vi "window_graph get_calc_region.vi"(9 "mouse up pos":cluster{"X":dbl, "Y":dbl}, 10 "mouse down pos":cluster{"X":dbl, "Y":dbl}, 11 "element":cluster{dbl[], sgl[]}) -> (1 "valid":bool, 2 "region data":cluster{"X":dbl, "Y":dbl}[](array[cluster]), 3 "limit data":cluster{"X":dbl, "Y":dbl}[](array[cluster]))   [LabVIEW 2018]
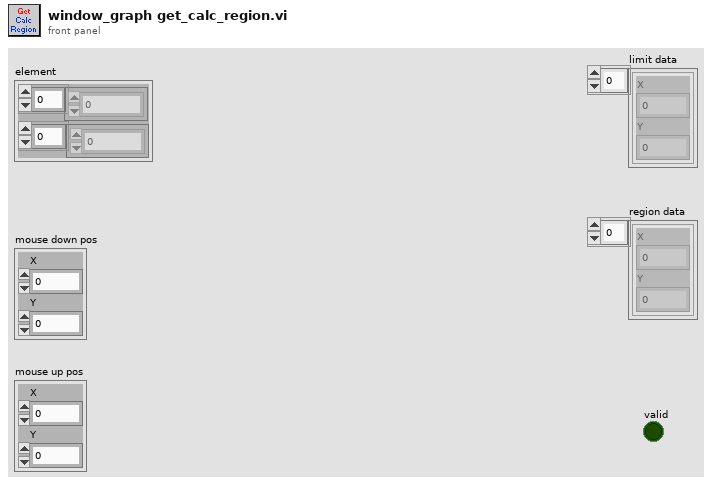
[diagram p1: front panel]
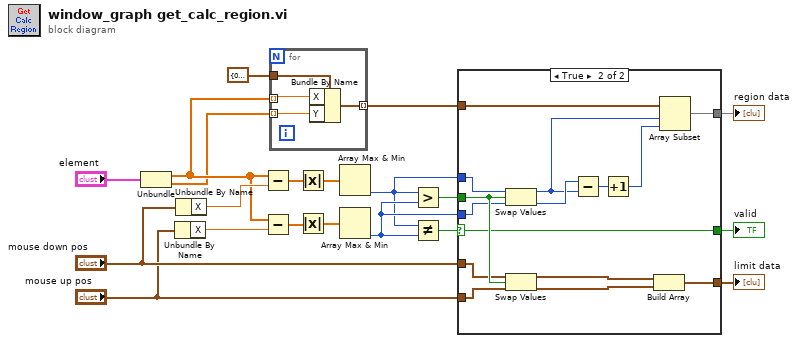
[diagram p0: block diagram]
diagram:
  n1 = Unbundle("element") -> (w13:dbl[], w12:sgl[])
  n2 = Unbundle By Name("mouse up pos") -> ("X"=w19:dbl)
  n3 = Unbundle By Name("mouse down pos") -> ("X"=w20:dbl)
  n4 = Subtract(x=w13, y=w20) -> (x-y=w18:dbl[])
  n5 = Subtract(x=w13, y=w19) -> (x-y=w17:dbl[])
  n6 = for {
    tunnel: cluster{"X":dbl, "Y":dbl} {"X"=0.0, "Y"=0.0} ("mouse down pos") -> [w24]
    tunnel: w13 -> [w23] mode=indexing
    tunnel: w12 -> [w22] mode=indexing
    tunnel: [w21] -> w4 mode=indexing
    n7 = Bundle By Name(cluster=w24, "X"=w23, "Y"=w22) -> (w21:cluster{"X":dbl, "Y":dbl})
  }
  n8 = Absolute Value(x=w18) -> (abs(x)=w16:dbl[])
  n9 = Absolute Value(x=w17) -> (abs(x)=w15:dbl[])
  n10 = Array Max & Min(array=w16) -> (min index (indices)=w5:i32)  [unwired: 3 out]
  n11 = Array Max & Min(array=w15) -> (min index (indices)=w6:i32)  [unwired: 3 out]
  n12 = Greater?(x=w5, y=w6) -> (0:w9:bool)
  n13 = Not Equal?(x=w5, y=w6) -> (x != y?=w10:bool)
  n14 = case shown="True" w10 {
    selector: w10 -> [w25 w30]
    tunnel: w9 -> [_ w40]
    tunnel: "mouse down pos" -> [_ w39]
    tunnel: "mouse up pos" -> [_ w38]
    tunnel: w6 -> [_ w36]
    tunnel: w5 -> [_ w37]
    tunnel: w4 -> [_ w29]
    tunnel: [_ w32] -> w1
    tunnel: [_ w31] -> w2
    tunnel: [w25 w30] -> w3
    frame False {
    }
    frame True {
      n15 = Swap Values(12:w37, 13:w40, 14:w36) -> (1:w28:i32, 3:w35:i32)
      n16 = Swap Values(12:w39, 13:w40, 14:w38) -> (1:w34:cluster{"X":dbl, "Y":dbl}, 3:w33:cluster{"X":dbl, "Y":dbl})
      n17 = Subtract(x=w35, y=w28) -> (x-y=w27:i32)
      n18 = Increment(x=w27) -> (x+1=w26:i32)
      n19 = Build Array(w34, w33) -> (w32:cluster{"X":dbl, "Y":dbl}[])
      n20 = Array Subset(array=w29, index=w28, length=w26) -> (w31:cluster{"X":dbl, "Y":dbl}[])
    }
  }
  "valid" <- w3
  "region data" <- w2
  "limit data" <- w1
